vi "START IT!.vi"() -> ()   [LabVIEW 2014]
doc: "Launches all the software required for data acquisition."
uses:
  Start all VIs Globals.vi
panel:
  in  "Stop":bool
  in  "User:":string
  in  "Existing File Location":path
  in  "Save this session's\n      parameters?":bool
  in  "Load existing file?":bool
  out "Starting Module Number:":u32(slide) scale=0.0..6.0
  out "Status":string="Ready"
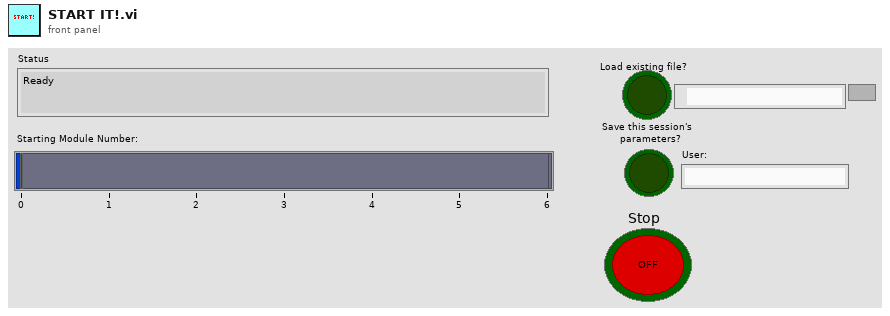
[diagram p1: front panel]
types:
  T1 = cluster{"VI Name":string, "Location":enum16{"TIRF Lock", "Camera & Acquisition VIs", "Stage Control", "Shutter Control"}, "Run?":bool, "Minimized?":bool, "Subdirectory (w trailing \"/\")":string}[]
  T2 = cluster{"Shutter Control":path, "Stage Control":path, "Camera & Acquisition VIs":path, "TIRF Lock":path}
  T3 = enum32{"Bad", "Idle", "Run top level", "Running"}
  T4 = enum32{"Invalid", "Standard", "Closed", "Hidden", "Minimized", "Maximized"}
  T5 = enum16{"TIRF Lock", "Camera & Acquisition VIs", "Stage Control", "Shutter Control"}
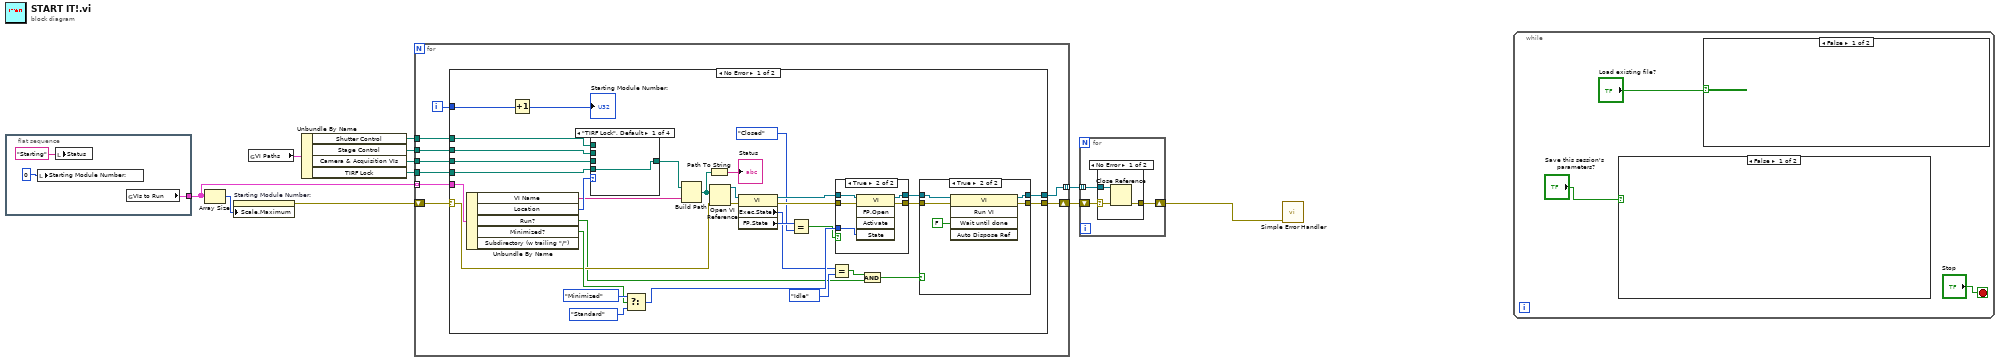
[diagram p0: block diagram]
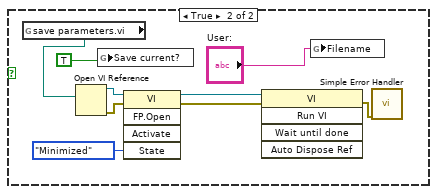
[diagram p2: hidden frame]
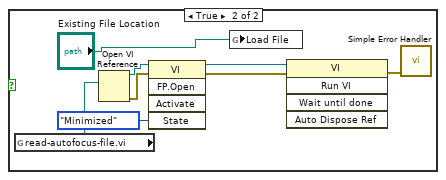
[diagram p3: hidden frame]
diagram:
  n1 = flat-sequence {
    tunnel: [w14] -> w2
    frame #0 {
      n2 = local write "Starting Module Number:"(0) -> ()
      n3 = local write "Status"("Starting") -> ()
      n4 = global read "Start all VIs Globals.vi" "VIs to Run"() -> (w14:T1)
    }
  }
  n5 = Array Size(array=w2) -> (size(s)=w3:i32)
  n6 = property on="Starting Module Number:" class="Slide (strict)"("Scale.Maximum"=w3) -> (error out=w4:errorcluster)  [unwired: 2 in, 1 out]
  n7 = global read "Start all VIs Globals.vi" "VI Paths"() -> (w11:T2)
  n8 = Unbundle By Name(w11) -> ("Shutter Control"=w10:path, "Stage Control"=w9:path, "Camera & Acquisition VIs"=w8:path, "TIRF Lock"=w7:path)
  n9 = for {
    tunnel: w10 -> [w22]
    tunnel: w9 -> [w21]
    tunnel: w8 -> [w20]
    tunnel: w7 -> [w19]
    tunnel: w2 -> [w23] mode=indexing
    tunnel: [w18] -> w6 mode=indexing
    shift-right: [w17] -> w5
    shift-left: w4 -> [w16]
    i -> [w15]
    n10 = case shown="No Error" w16 {
      selector: w16 -> [w44 w75]
      tunnel: w23 -> [w56 _]
      tunnel: w22 -> [w54 _]
      tunnel: w21 -> [w53 _]
      tunnel: w20 -> [w52 _]
      tunnel: w19 -> [w51 _]
      tunnel: [w25 _] -> w18
      tunnel: [w24 w75] -> w17
      tunnel: w15 -> [w42 _]
      frame No Error {
        n11 = Unbundle By Name(w56) -> ("VI Name"=w49:string, "Location"=w55:T5, "Run?"=w29:bool, "Minimized?"=w46:bool)  [unwired: 1 out]
        n12 = Increment(x=w42) -> (x+1=→"Starting Module Number:":i32)
        n13 = case shown="\"TIRF Lock\", Default" w55 {
          tunnel: w54 -> [_ _ _ w74]
          tunnel: w53 -> [_ _ w73 _]
          tunnel: w52 -> [_ w72 _ _]
          tunnel: w51 -> [w71 _ _ _]
          tunnel: [w71 w72 w73 w74] -> w50
          frame "TIRF Lock", Default {
          }
          frame "Camera & Acquisition VIs" {
          }
          frame "Stage Control" {
          }
          frame "Shutter Control" {
          }
        }
        n14 = Select(t=T4."Minimized" ("State"), s=w46, f=T4."Standard" ("State")) -> (s? t:f=w45:T4)
        n15 = Build Path(base path=w50, name or relative path=w49) -> (appended path=w40:path)
        n16 = Path To String(path=w40) -> (string=→"Status":string)
        n17 = Open VI Reference(vi path=w40, error in (no error)=w44) -> (vi reference=w38:refnum<vi>, error out=w39:errorcluster)  [unwired: 4 out]
        n18 = property class="VI"(reference=w38, error in=w39) -> (reference out=w36:refnum<vi>, error out=w37:errorcluster, "Exec.State"=w32:T3, "FP.State"=w35:T4)
        n19 = Equal?(x=w35, y=T4."Closed" ("State")) -> (x = y?=w33:bool)
        n20 = Equal?(x=w32, y=T3."Idle") -> (x = y?=w30:bool)
        n21 = case shown="True" w33 {
          tunnel: w36 -> [w64 w70]
          tunnel: w37 -> [w65 w69]
          tunnel: w45 -> [_ w68]
          tunnel: [w64 w67] -> w26
          tunnel: [w65 w66] -> w27
          frame False {
          }
          frame True {
            n22 = invoke class="VI" method="FP.Open"(reference=w70, error in=w69, "State"=w68) -> (reference out=w67:refnum<vi>, error out=w66:errorcluster)  [unwired: 2 in, 3 out]
          }
        }
        n23 = And(x=w30, y=w29) -> (x .and. y?=w28:bool)
        n24 = case shown="True" w28 {
          tunnel: w27 -> [w58 w61]
          tunnel: w26 -> [w57 w62]
          tunnel: [w57 w60] -> w25
          tunnel: [w58 w59] -> w24
          frame False {
          }
          frame True {
            n25 = invoke class="VI" method="Run VI"(reference=w62, error in=w61, "Wait until done"=FALSE ("Wait Until Done")) -> (reference out=w60:refnum<vi>, error out=w59:errorcluster)  [unwired: 2 in, 3 out]
          }
        }
      }
      frame Error {
      }
    }
  }
  n26 = for {
    tunnel: w6 -> [w78] mode=indexing
    shift-right: [w77] -> w1
    shift-left: w5 -> [w76]
    n27 = case shown="No Error" w76 {
      selector: w76 -> [w81 w82]
      tunnel: w78 -> [w80 _]
      tunnel: [w79 w82] -> w77
      frame No Error {
        n28 = Close Reference(reference=w80, error in (no error)=w81) -> (error out=w79:errorcluster)
      }
      frame Error {
      }
    }
  }
  n29 = call <vilib>:"Simple Error Handler.vi"("error in (no error)"=w1) -> ()  [unwired: 4 in, 5 out]
  n30 = while {
    stop <- "Stop" stop-if-true
    n31 = case shown="False" "Save this session's\n      parameters?" {
      frame False {
      }
      frame True {
        n32 = global read "Start all VIs Globals.vi" "save parameters.vi"() -> (w88:path)
        n33 = Open VI Reference(vi path=w88) -> (vi reference=w90:refnum<vi>, error out=w89:errorcluster)  [unwired: 1 in, 4 out]
        n34 = global write "Start all VIs Globals.vi" "Save current?"(TRUE) -> ()
        n35 = invoke class="VI" method="FP.Open"(reference=w90, error in=w89, "State"=T4."Minimized") -> (reference out=w92:refnum<vi>, error out=w93:errorcluster)  [unwired: 2 in, 3 out]
        n36 = invoke class="VI" method="Run VI"(reference=w92, error in=w93) -> (error out=w91:errorcluster)  [unwired: 3 in, 4 out]
        n37 = global write "Start all VIs Globals.vi" "Filename"("User:") -> ()
        n38 = call <vilib>:"Simple Error Handler.vi"("error in (no error)"=w91) -> ()  [unwired: 4 in, 5 out]
      }
    }
    n39 = case shown="False" "Load existing file?" {
      frame False {
      }
      frame True {
        n40 = global read "Start all VIs Globals.vi" "read-autofocus-file.vi"() -> (w96:path)
        n41 = Open VI Reference(vi path=w96) -> (vi reference=w97:refnum<vi>, error out=w98:errorcluster)  [unwired: 1 in, 4 out]
        n42 = invoke class="VI" method="FP.Open"(reference=w97, error in=w98, "State"=T4."Minimized") -> (reference out=w100:refnum<vi>, error out=w101:errorcluster)  [unwired: 2 in, 3 out]
        n43 = global write "Start all VIs Globals.vi" "Load File"("Existing File Location") -> ()
        n44 = invoke class="VI" method="Run VI"(reference=w100, error in=w101) -> (error out=w99:errorcluster)  [unwired: 3 in, 4 out]
        n45 = call <vilib>:"Simple Error Handler.vi"("error in (no error)"=w99) -> ()  [unwired: 4 in, 5 out]
      }
    }
  }
